vi "filter -- balance logic.vi"(8 "tale of three indices":T1={"left"=0, "center"=0, "right"=0, "right most"=0, "left most"=0, "window"=0, "max win factor"=2, "max win"=2, "min win"=2}, 10 "span":dbl, 11 "Array":cdb[](array[numeric])) -> (0 "three indices out":T1={"left"=0, "center"=0, "right"=0, "right most"=0, "left most"=0, "window"=0, "max win factor"=2, "max win"=2, "min win"=2}, 1 "center out":cdb, 2 "span out":dbl, 3 "Array out":cdb[](array[numeric]))   [LabVIEW 2018]
uses:
  tale of three indices -- int -- control.ctl
  tale of three indices -- selector -- control.ctl
  Q - not nan -- real.vi
  command stack.vi
  tale of three indices -- check state.vi
  Q -- check range -- i -- integer.vi
  Q - not nan -- integer.vi
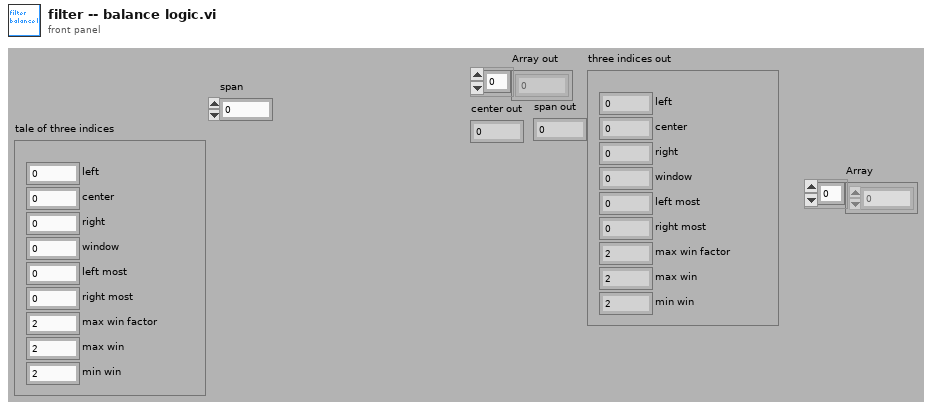
[diagram p1: front panel]
types:
  T1 = typedef "tale of three indices -- int -- control.ctl" = cluster{"left":i32, "center":i32, "right":i32, "right most":i32, "left most":i32, "window":i32, "max win factor":i32, "max win":i32, "min win":i32}
  T2 = typedef "tale of three indices -- selector -- control.ctl" = enum16{"window right", "window left", "balance", "shrink", "grow", "do nothing", "reset", "center right", "center left", "all left", "all right", "right wing shrink", "left wing shrink", "left wing grow", "right wing grow", "skew left", "skew right", "check"}
  T3 = typedef "comparison control.ctl" = enum16{"not a number", "above", "in range", "below"}
  T4 = typedef "comparison control - double.ctl" = enum16{"both above", "both below", "both in range", "above , below", "below, above", "other"}
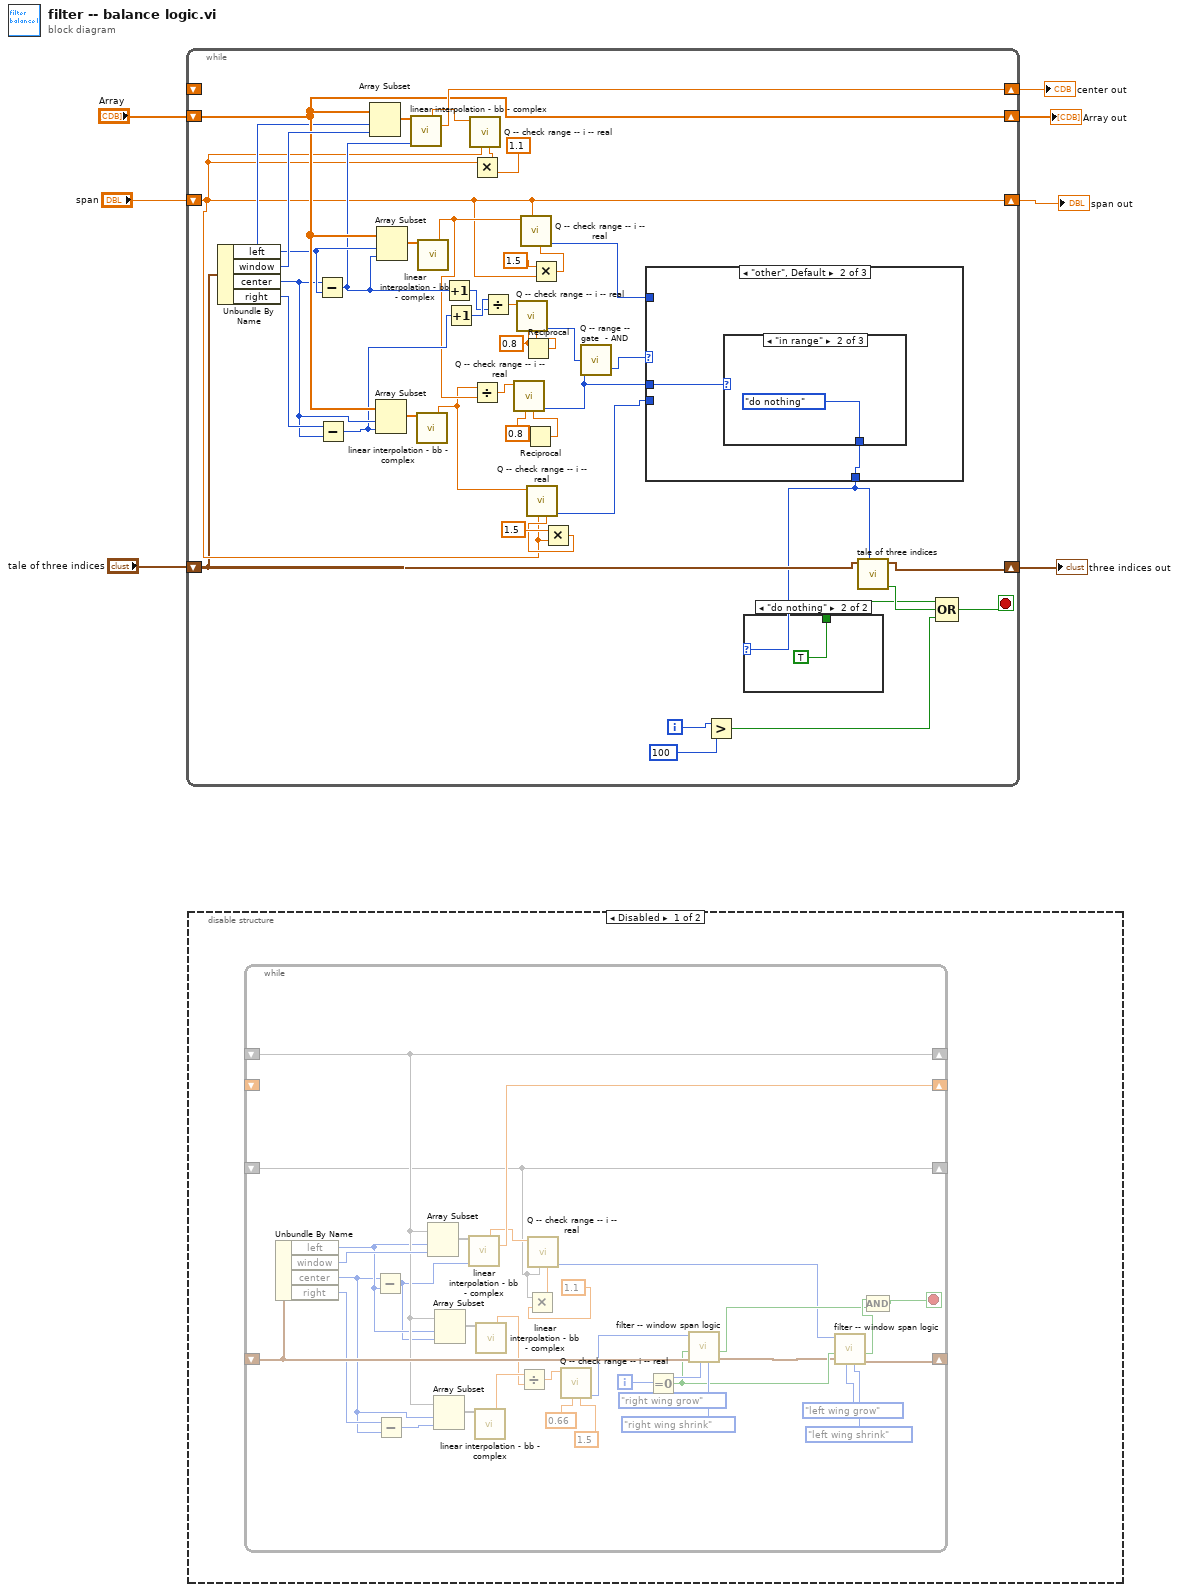
[diagram p0: block diagram]
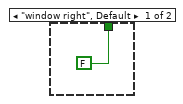
[diagram p3: hidden frame]
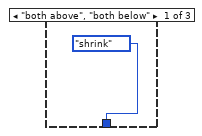
[diagram p4: hidden frame]
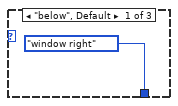
[diagram p5: hidden frame]
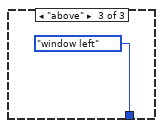
[diagram p6: hidden frame]
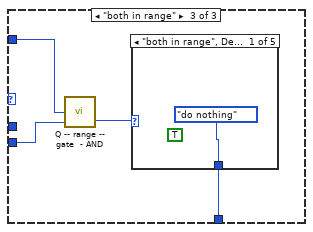
[diagram p7: hidden frame]
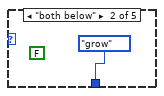
[diagram p8: hidden frame]
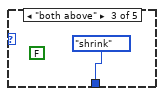
[diagram p9: hidden frame]
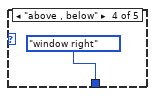
[diagram p10: hidden frame]
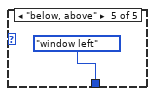
[diagram p11: hidden frame]
diagram:
  n1 = while {
    shift-right: [w19] -> w1
    shift-left: "tale of three indices" -> [w20]
    shift-right: [w49] -> w3
    shift-left: _ -> [_]
    shift-right: [w45] -> w4
    shift-left: "Array" -> [w45]
    shift-right: [w21] -> w2
    shift-left: "span" -> [w21]
    i -> [w14]
    stop <- w17 stop-if-true
    w31 = 0.8 ("y")
    w30 = 0.8 ("y")
    n2 = Unbundle By Name(w20) -> ("left"=w44:i32, "window"=w48:i32, "center"=w42:i32, "right"=w43:i32)
    n3 = Subtract(x=w42, y=w44) -> (x-y=w37:i32)
    n4 = Subtract(x=w43, y=w42) -> (x-y=w36:i32)
    n5 = Array Subset(array=w45, index=w44, length=w48) -> (w50:cdb[])
    n6 = Array Subset(array=w45, index=w42, length=w36) -> (w46:cdb[])
    n7 = Array Subset(array=w45, index=w44, length=w37) -> (w47:cdb[])
    n8 = call "linear interpolation - bb - complex.vi"("Array"=w50, "center"=w37) -> ("directed sigma"=w41:dbl, "center"=w49:cdb)  [unwired: 5 in, 7 out]
    n9 = call "linear interpolation - bb - complex.vi"("Array"=w46) -> ("directed sigma"=w23:dbl)  [unwired: 6 in, 8 out]
    n10 = call "linear interpolation - bb - complex.vi"("Array"=w47) -> ("directed sigma"=w28:dbl)  [unwired: 6 in, 8 out]
    n11 = Increment(x=w37) -> (x+1=w34:i32)
    n12 = Increment(x=w36) -> (x+1=w35:i32)
    n13 = Multiply(x=w21, y=1.1) -> (x*y=w38:dbl)
    n14 = call "Q -- check range -- i -- real.vi"("upper"=w38, "lower"=w21, "number"=w41) -> ()  [unwired: 6 in, 3 out]
    n15 = Divide(x=w23, y=w28) -> (x/y=w40:dbl)
    n16 = Divide(x=w35, y=w34) -> (x/y=w33:dbl)
    n17 = Reciprocal(x=w31) -> (1/x=w32:dbl)
    n18 = call "Q -- check range -- i -- real.vi"("upper"=w32, "lower"=w31, "number"=w33) -> ("selector"=w11:T3)  [unwired: 6 in, 2 out]
    n19 = Reciprocal(x=w30) -> (1/x=w29:dbl)
    n20 = call "Q -- check range -- i -- real.vi"("upper"=w29, "lower"=w30, "number"=w40) -> ("selector"=w8:T3)  [unwired: 6 in, 2 out]
    n21 = Multiply(x=1.5, y=w21) -> (x*y=w26:dbl)
    n22 = call "Q -- check range -- i -- real.vi"("upper"=w26, "lower"=w21, "number"=w28) -> ("selector"=w22:T3)  [unwired: 6 in, 2 out]
    n23 = Multiply(x=1.5, y=w21) -> (x*y=w24:dbl)
    n24 = call "Q -- check range -- i -- real.vi"("upper"=w24, "lower"=w21, "number"=w23) -> ("selector"=w10:T3)  [unwired: 6 in, 2 out]
    n25 = call "Q -- range -- gate  - AND.vi"("state two"=w8, "state one"=w11) -> ("selector"=w9:T4)  [unwired: 3 in]
    n26 = case shown="\"other\", Default" w9 {
      tunnel: w22 -> [_ _ w62]
      tunnel: w10 -> [_ _ w61]
      tunnel: [tale_of_three_indices_--_selector_--_control."shrink" ("selector") w55 w60] -> w16
      tunnel: w8 -> [_ w54 _]
      frame "both above", "both below" {
      }
      frame "other", Default {
        n27 = case shown="\"in range\"" w54 {
          tunnel: [tale_of_three_indices_--_selector_--_control."window right" ("selector") tale_of_three_indices_--_selector_--_control."do nothing" ("selector") tale_of_three_indices_--_selector_--_control."window left" ("selector")] -> w55
          frame "below", Default {
          }
          frame "in range" {
          }
          frame "above" {
          }
        }
      }
      frame "both in range" {
        n28 = call "Q -- range -- gate  - AND.vi"("state two"=w61, "state one"=w62) -> ("selector"=w59:T4)  [unwired: 3 in]
        n29 = case shown="\"both in range\", Default" w59 {
          tunnel: [tale_of_three_indices_--_selector_--_control."do nothing" ("selector") tale_of_three_indices_--_selector_--_control."grow" ("selector") tale_of_three_indices_--_selector_--_control."shrink" ("selector") tale_of_three_indices_--_selector_--_control."window right" ("selector") tale_of_three_indices_--_selector_--_control."window left" ("selector")] -> w60
          frame "both in range", Default {
            (unwired) TRUE
          }
          frame "both below" {
            (unwired) FALSE
          }
          frame "both above" {
            (unwired) FALSE
          }
          frame "above , below" {
          }
          frame "below, above" {
          }
        }
      }
    }
    n30 = Greater?(x=w14, y=100) -> (0:w12:bool)
    n31 = case shown="\"do nothing\"" w16 {
      tunnel: [FALSE TRUE] -> w15
      frame "window right", Default {
      }
      frame "do nothing" {
      }
    }
    n32 = call "tale of three indices.vi"("selector"=w16, "tale of three indices -- int -- control"=w20) -> ("no success ?"=w18:bool, "tale of three indices -- int -- control out"=w19:T1)  [unwired: 6 in, 2 out]
    n33 = Compound Arithmetic op=OR(w15, w18, w12) -> (w17:bool)
  }
  "Array out" <- w4
  "center out" <- w3
  "span out" <- w2
  "three indices out" <- w1
  n34 = disable-structure shown="Disabled" {
    frame Disabled {
      n35 = while {
        shift-right: [w81] -> _
        shift-left: _ -> [w98]
        shift-right: [w100] -> _
        shift-left: _ -> [_]
        shift-right: [w92] -> _
        shift-left: _ -> [w92]
        shift-right: [w73] -> _
        shift-left: _ -> [w73]
        i -> [w97]
        stop <- w80 stop-if-true
        n36 = Unbundle By Name(w98) -> ("left"=w91:i32, "window"=w99:i32, "center"=w88:i32, "right"=w89:i32)
        n37 = Subtract(x=w88, y=w91) -> (x-y=w90:i32)
        n38 = Subtract(x=w89, y=w88) -> (x-y=w87:i32)
        n39 = Array Subset(array=w92, index=w91, length=w99) -> (w101:void[])
        n40 = Array Subset(array=w92, index=w88, length=w87) -> (w93:void[])
        n41 = Array Subset(array=w92, index=w91, length=w90) -> (w94:void[])
        n42 = call "linear interpolation - bb - complex.vi"("Array"=w101, "center"=w90) -> ("directed sigma"=w86:dbl, "center"=w100:cdb)  [unwired: 5 in, 7 out]
        n43 = call "linear interpolation - bb - complex.vi"("Array"=w93) -> ("directed sigma"=w84:dbl)  [unwired: 6 in, 8 out]
        n44 = call "linear interpolation - bb - complex.vi"("Array"=w94) -> ("directed sigma"=w83:dbl)  [unwired: 6 in, 8 out]
        n45 = Divide(x=w84, y=w83) -> (x/y=w85:dbl)
        n46 = Multiply(x=w73, y=1.1) -> (x*y=w71:dbl)
        n47 = call "Q -- check range -- i -- real.vi"("upper"=w71, "lower"=w73, "number"=w86) -> ("selector"=w74:T3)  [unwired: 6 in, 2 out]
        n48 = call "Q -- check range -- i -- real.vi"("upper"=1.5 ("y"), "lower"=0.66 ("y"), "number"=w85) -> ("selector"=w69:T3)  [unwired: 6 in, 2 out]
        n49 = Equal To 0?(x=w97) -> (x = 0?=w70:bool)
        n50 = call "filter -- window span logic.vi"("action for \"above\""=tale_of_three_indices_--_selector_--_control."right wing shrink" ("selector"), "action for \"below\""=tale_of_three_indices_--_selector_--_control."right wing grow" ("selector"), "tale of three indices -- int -- control out"=w98, "start"=w70, "new state"=w69) -> ("three indices out"=w68:T1, "stop"=w78:bool)  [unwired: 5 in]
        n51 = call "filter -- window span logic.vi"("action for \"above\""=tale_of_three_indices_--_selector_--_control."left wing shrink" ("selector"), "action for \"below\""=tale_of_three_indices_--_selector_--_control."left wing grow" ("selector"), "tale of three indices -- int -- control out"=w68, "start"=w70, "new state"=w74) -> ("three indices out"=w81:T1, "stop"=w79:bool)  [unwired: 5 in]
        n52 = Compound Arithmetic op=AND(w79, w78) -> (w80:bool)
      }
    }
    frame Enabled {
    }
  }
